vi "PV Handheld Data Logging.vi"(8 "error in (no error)":errorcluster, 9 "Handheld Gauge Data Logging-Cluster":T1 {"Data logging interval" max=9999 step=1; "Parameter" items=[" Data logging interval [s]", " Data logging record (read only)"]}, 10 "Adress of unit":u16=1 max=999 step=1, 11 "VISA session":refnum<visa-resource-name>) -> (0 "error out":errorcluster, 2 "response (data)":string, 3 "dup VISA session":refnum<visa-resource-name>)   [LabVIEW 2016, in "Pfeiffer Vacuum.lvlib"]
doc: "There are 2 parameters available, only one of which can be enabled at a time. \n\n0 - Data logging interval [s] (default)\n1 - Data logging record (read only)\n\nNote: The 1 control right of this one will set the appropriate values for the selected parameter. Any settings for an parameter that is not selected will be ignored. If a value is out of range, it will be changed to either the upper or the lower limit of the range."
uses:
  Pfeiffer Vacuum.lvlib
  Handheld Gauge Data Logging - Cluster.ctl
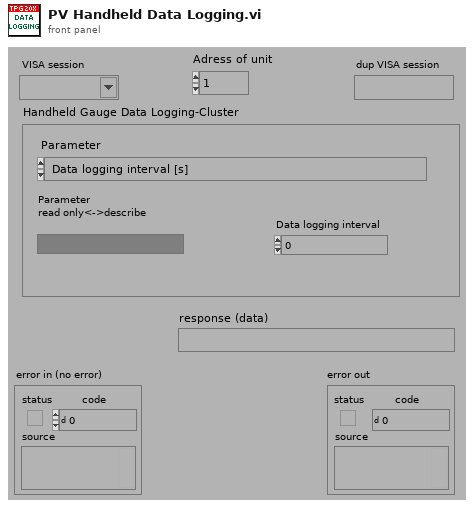
[diagram p1: front panel]
types:
  T1 = typedef "Pfeiffer Vacuum.lvlib/Handheld Gauge Data Logging - Cluster.ctl" = cluster{"Parameter":u16, "Parameter\nread only<->describe":bool, "Data logging interval":u16}
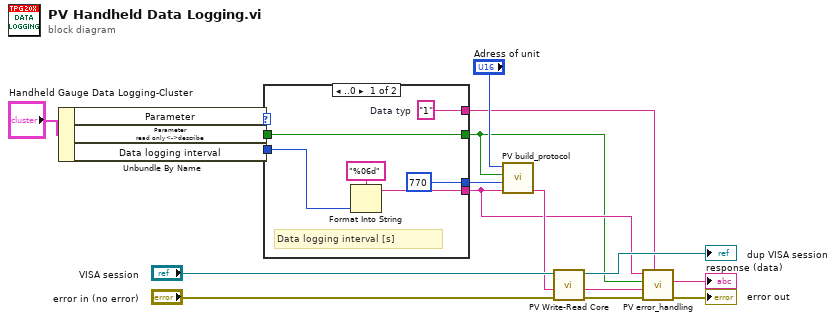
[diagram p0: block diagram]
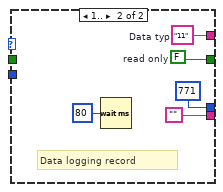
[diagram p2: hidden frame]
diagram:
  n1 = Unbundle By Name("Handheld Gauge Data Logging-Cluster") -> ("Parameter"=w15:u16, "Parameter\nread only<->describe"=w14:bool, "Data logging interval"=w3:u16)
  n2 = case shown="..0" w15 {
    tunnel: [u16 770 ("Parameter-number") u16 771 ("Parameter-number")] -> w16
    tunnel: [w18 ""] -> w6
    tunnel: [w21 w26] -> w5
    tunnel: w14 -> [w21 _]
    tunnel: [w22 w27] -> w7
    tunnel: w3 -> [w19 _]
    frame ..0 {
      w22 = "1"  # Data typ
      # "Data logging interval [s]"
      n3 = Format Into String(format string="%06d" ("Format-String"), w19) -> (resulting string=w18:string)  [unwired: 2 in, 1 out]
    }
    frame 1.. {
      w26 = FALSE  # read only
      w27 = "11"  # Data typ
      # "Data logging record"
      n4 = Wait (ms)(milliseconds to wait=u32 80 ("Zu wartende ms")) -> ()  [unwired: 1 out]
    }
  }
  n5 = call "PV build_protocol.vi"("Data"=w6, "Parameter-number"=w16, "parameter\nread<->describe"=w5, "Adress"="Adress of unit") -> ("output"=w10:string)  [unwired: 3 in]
  n6 = call "PV Write-Read Core.vi"("error in"="error in (no error)", "Write data in"=w10, "VISA session"="VISA session") -> ("error out"=w8:errorcluster, "response (data) out"=w1:string, "dup VISA session"=→"dup VISA session":refnum<visa-resource-name>)  [unwired: 2 in]
  n7 = call "PV error_handling.vi"("Data Typ in"=w7, "error in"=w8, "response (data) in"=w1, "Parameter\nread only<->describe"=w5, "data in"=w6) -> ("error out"=→"error out":errorcluster, "Data out"=→"response (data)":string)  [unwired: 4 in, 1 out]
